vi "Add Icons From Paths.vi"(8 "error in (no error)":errorcluster, 9 "Names":string[](array[string]), 10 "Paths":path[](array[path]), 11 "Toolbar Control in":refnum<class "Toolbar Control.lvclass">) -> (0 "error out":errorcluster, 3 "Toolbar Control out":refnum<class "Toolbar Control.lvclass">)   [LabVIEW 2011, in "Toolbar Control.lvclass"]
doc: "This VI will add the image <B>Image Paths</B> to the <B>Toolbar Control in</B> at the available location or if specified by <B>Icon Index (Next)</B>. The name of the button will default to the file name or one provided by <B>Icon Names</B>. The image file can be a PNG with alpha layers.\n\n-------------\nDeveloped by Brian Hoover (hooovahh)"
uses:
  Toolbar Control.lvclass
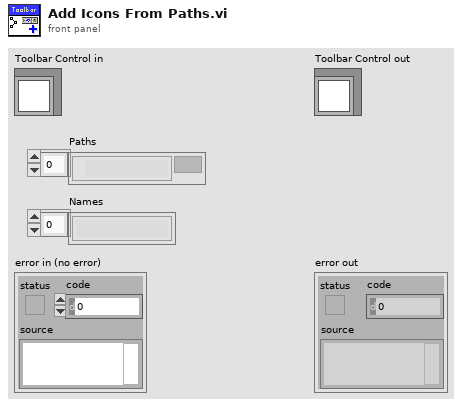
[diagram p1: front panel]
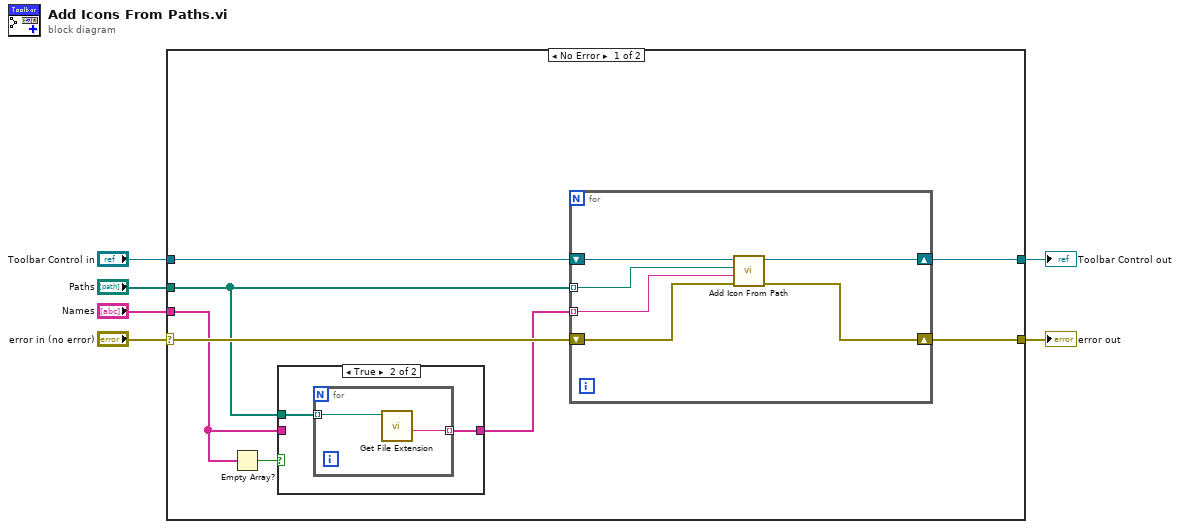
[diagram p0: block diagram]
diagram:
  n1 = case shown="No Error" "error in (no error)" {
    selector: "error in (no error)" -> [w12 w27]
    tunnel: [w11 w27] -> w5
    tunnel: [w13 w26] -> w3
    tunnel: "Toolbar Control in" -> [w14 w26]
    tunnel: "Paths" -> [w9 _]
    tunnel: "Names" -> [w8 _]
    frame No Error {
      n2 = Empty Array?(array=w8) -> (empty?=w10:bool)
      n3 = case shown="True" w10 {
        tunnel: w9 -> [_ w17]
        tunnel: [w15 w16] -> w7
        tunnel: w8 -> [w15 _]
        frame False {
        }
        frame True {
          n4 = for {
            tunnel: w17 -> [w19] mode=indexing
            tunnel: [w18] -> w16 mode=indexing
            n5 = call <vilib>:"Get File Extension.vi"("file"=w19) -> ("filename without extension"=w18:string)  [unwired: 7 in, 3 out]
          }
        }
      }
      n6 = for {
        tunnel: w9 -> [w23] mode=indexing
        shift-right: [w24] -> w13
        shift-left: w14 -> [w25]
        tunnel: w7 -> [w22] mode=indexing
        shift-right: [w20] -> w11
        shift-left: w12 -> [w21]
        n7 = call "Add Icon From Path.vi"("error in (no error)"=w21, "Icon Name"=w22, "Image Path"=w23, "Toolbar Control in"=w25) -> ("error out"=w20:errorcluster, "Toolbar Control out"=w24:refnum<class "Toolbar Control.lvclass">)  [unwired: 6 in]
      }
    }
    frame Error {
    }
  }
  "error out" <- w5
  "Toolbar Control out" <- w3
